vi "VISAandHTTTPconnection.vi"() -> ()   [LabVIEW 2020]
uses:
  <vilib>/httpClient/PUTBuffer.vi
  <vilib>/httpClient/LabVIEWHTTPClient.lvlib
panel:
  in  "IR and Force Sensor":bool
  in  "Train Speed":dbl
  in  "Trolley Speed":dbl
  in  "Trolley Distance":dbl
  in  "Elephant Distance":dbl
  out "error out":errorcluster
  in  "stop":bool
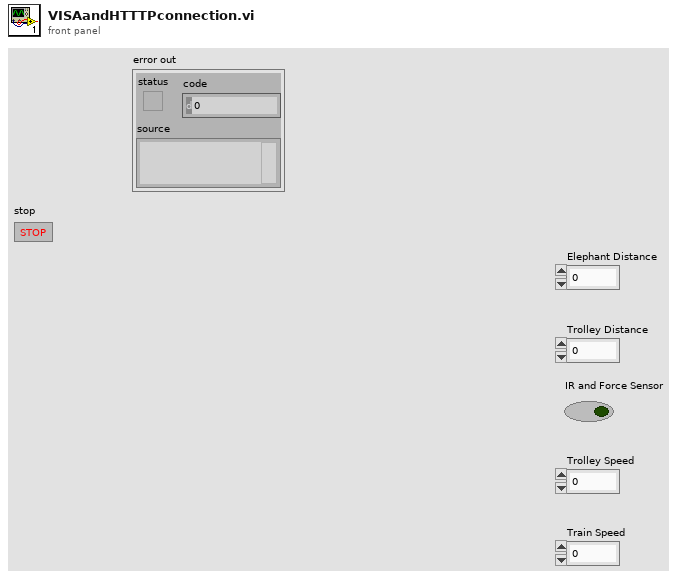
[diagram p1: front panel]
types:
  T1 = typedef "LabVIEWHTTPClient.lvlib/ClientHandle.ctl" = refnum<k1>
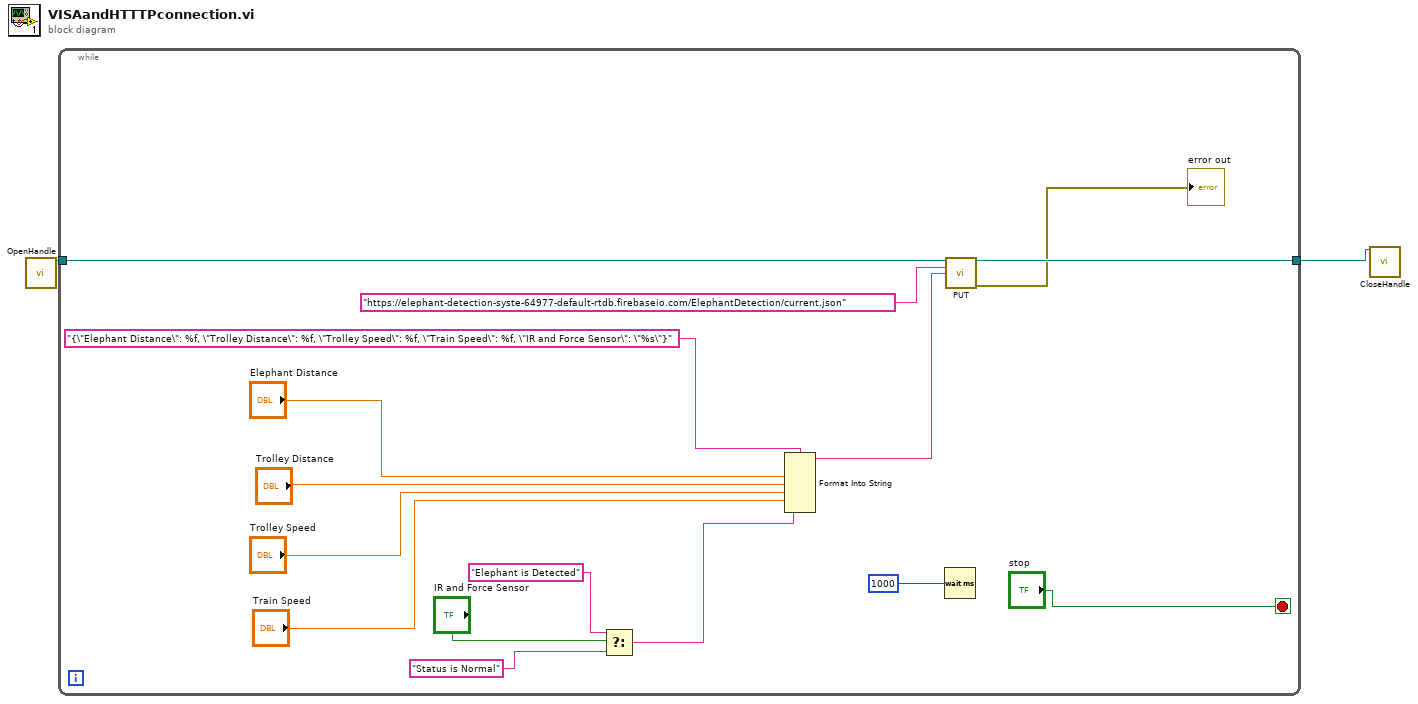
[diagram p0: block diagram]
diagram:
  n1 = call <vilib>:"OpenHandle.vi"() -> ("client handle out"=w2:T1)  [unwired: 14 in, 1 out]
  n2 = while {
    tunnel: w2 -> [w16]
    tunnel: [w14] -> w1
    stop <- "stop" stop-if-true
    n3 = Select(t="Elephant is Detected" ("format string"), s="IR and Force Sensor", f="Status is Normal" ("format string")) -> (s? t:f=w5:string)
    n4 = Format Into String(format string="{\"Elephant Distance\": %f, \"Trolley Distance\": %f, \"Trolley Speed\": %f, \"Train Speed\": %f, \"IR and Force Sensor\": \"%s\"}", "Elephant Distance", "Trolley Distance", "Trolley Speed", "Train Speed", w5) -> (resulting string=w3:string)  [unwired: 2 in, 1 out]
    n5 = Wait (ms)(milliseconds to wait=1000) -> ()  [unwired: 1 out]
    n6 = call-poly <vilib>:"PUT.vi"("client handle"=w16, "url"="https://elephant-detection-syste-64977-default-rtdb.firebaseio.com/ElephantDetection/current.json", "buffer"=w3) -> ("client handle out"=w14:T1, "error out"=→"error out":errorcluster)  [unwired: 9 in, 2 out]
  }
  n7 = call <vilib>:"CloseHandle.vi"("client handle"=w1) -> ()  [unwired: 14 in, 1 out]
